vi "Lockin Take Data - Outputs.vi"(8 "error in (no error)":errorcluster caption="Error in (no error)") -> (0 "output2":dbl format="%#_12g", 1 "output1":dbl format="%#_12g", 2 "output2":string, 3 "output1":string, 4 "error out":errorcluster caption="Error")   [LabVIEW 2017, in "SR830.lvlib"]
doc: "Reads the values currently displayed on the front panel of the lock-in detector."
uses:
  SR830.lvlib
  Global/GPIB Numbers.vi
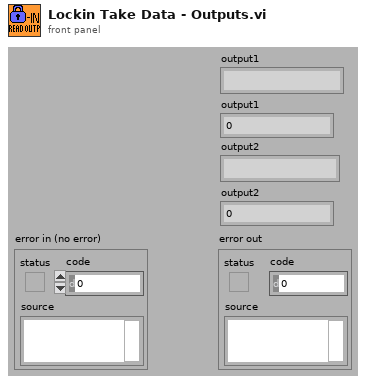
[diagram p1: front panel]
types:
  T1 = typedef "GPIB Type Def.ctl" = cluster{"Name":string, "bus":dbl, "GPIB":dbl, "GPIB as string":string, "byte":i32, "VISA Resource Name":refnum<visa-resource-name>}
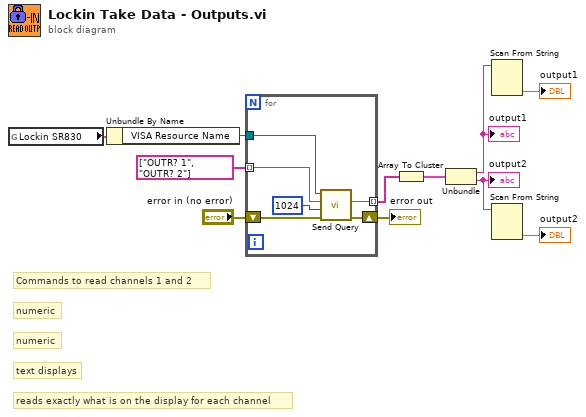
[diagram p0: block diagram]
diagram:
  # "Commands to read channels 1 and 2"
  # "numeric"
  # "numeric"
  # "text displays"
  # "reads exactly what is on the display for each channel"
  n1 = global read "GPIB Numbers.vi" "Lockin SR830"() -> (w3:T1)
  n2 = Unbundle By Name(w3) -> ("VISA Resource Name"=w2:refnum<visa-resource-name>)
  n3 = for {
    tunnel: [w13] -> w8 mode=indexing
    shift-right: [w12] -> w11
    shift-left: "error in (no error)" -> [w17]
    tunnel: w2 -> [w14]
    tunnel: string[] ["OUTR? 1", "OUTR? 2"] -> [w15] mode=indexing
    n4 = call "Send Query.vi"("error in (no error)"=w17, "Bytes Count"=1024, "write buffer"=w15, "VISA resource name"=w14) -> ("error out"=w12:errorcluster, "read buffer"=w13:string)  [unwired: 5 in, 1 out]
  }
  "error out" <- w11
  n5 = Array To Cluster(array=w8) -> (cluster=w9:cluster{"[0]":string, "[1]":string})
  n6 = Unbundle(w9) -> ("[0]"=w7:string, "[1]"=w6:string)
  "output1" <- w7
  "output2" <- w6
  n7 = Scan From String(input string=w7) -> (output 1=→"output1":dbl)  [unwired: 3 in, 4 out]
  n8 = Scan From String(input string=w6) -> (output 1=→"output2":dbl)  [unwired: 3 in, 4 out]
